vi "cmd_set_speed.vi"(8 "error in (no error)":errorcluster, 11 "JSON":string) -> (0 "error out":errorcluster)   [LabVIEW 2021]
doc: "Set the maximum change in analogue output per output.\n \n :param speed: Specifies the maximum changes (8ch)"
uses:
  core/host_global_vars.vi
  <vilib>/Utility/error.llb/Error Cluster From Error Code.vi
  <vilib>/rvi/errors/niLvFpgaAdjustHostInterfaceError.vi
  <vilib>/rvi/interface/nirviReadWriteControl/nirviReadWriteControl.xnode
  fpga/fpga_dtype_sgl_8ch.ctl
  FPGA Bitfiles/openlabspm_FPGATarget_fpgamain_eo-gUZR5D1g.lvbitx
  fpga/fpga_main.vi
  NiFpgaLv.dll
panel:
  in  "args":cluster{"speed":sgl[]}
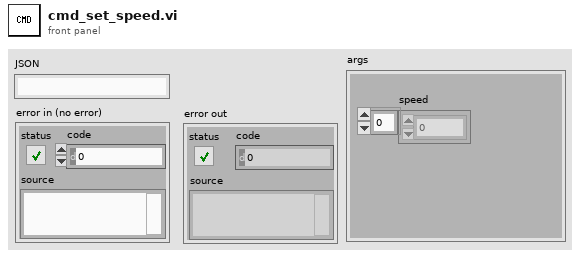
[diagram p1: front panel]
types:
  T1 = cluster{"speed[0]":sgl, "speed[1]":sgl, "speed[2]":sgl, "speed[3]":sgl, "speed[4]":sgl, "speed[5]":sgl, "speed[6]":sgl, "speed[7]":sgl}
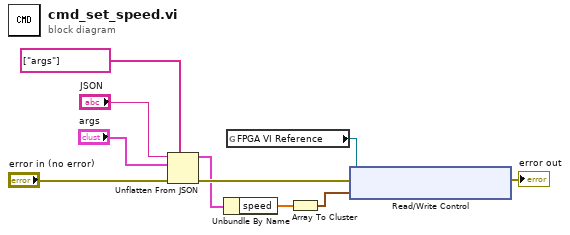
[diagram p0: block diagram]
diagram:
  n1 = Unflatten From JSON(path=string[] ["args"], JSON string="JSON", type and defaults="args", error in (no error)="error in (no error)") -> (value=w4:cluster{"speed":sgl[]}, error out=w5:errorcluster)  [unwired: 3 in]
  n2 = Unbundle By Name(w4) -> ("speed"=w2:sgl[])
  n3 = global read "host_global_vars.vi" "FPGA VI Reference"() -> (w6:refnum<k20>)
  n4 = Array To Cluster(array=w2) -> (cluster=w1:T1)
  n5 = xnode "Read/Write Control"("FPGA VI Reference In"=w6, "error in"=w5, "speed"=w1) -> ("error out"=→"error out":errorcluster)  [unwired: 1 out]
